vi "Tower_lamp.vi"(10 "DOs":bool[](array[boolean])=[TRUE, FALSE, FALSE, FALSE], 11 "Relay_Channel_OUT":T1[](array[typedef])) -> ()   [LabVIEW 2024, in "ADAM_DI.lvlib"]
uses:
  ADAM_DI.lvlib
  Relay_Enum_OUT.ctl
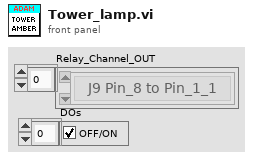
[diagram p1: front panel]
types:
  T1 = typedef "ADAM_DI.lvlib/Relay_Enum_OUT.ctl" = enum16{"J9 Pin_8 to Pin_1_1", "J9 Pin_8 to Pin_1_2", "J9 Pin_7 to Pin_1_1", "J9 Pin_7 to Pin_1_2", "J9 Pin_8 to Pin_7_1", "J9 Pin_8 to Pin_7_2", "J9 Pin_5 to Pin_1_1", "J9 Pin_5 to Pin_1_2", "J9 Pin_6 to Pin_1_1", "J9 Pin_6 to Pin_1_2", "J9 Pin_4 to Pin_1_1", "J9 Pin_4 to Pin_1_2", "J9 Pin_3 to Pin_1_1", "J9 Pin_3 to Pin_1_2", "PS(GND) to Pin1_1 J9", "PS(GND) to Pin1_2 J9", "PS(+14V) to Pin_3_1", "PS(+14V) to Pin_3_2", "PS(+12V) to Pin_4_1_ J9", "PS(+12V) to Pin_4_2_ J9", "PS(+12V) to Pin_5_1 J9", "PS(+12V) to Pin_5_2 J9", "PS(+12V) to Pin_6_1 J9", "PS(+12V) to Pin_6_2 J9", "Tower Amber", "Tower Red", "Tower Green", "Tower Buzzer", "PS(GND) to TP3_1", "PS(GND) to TP3_2", "PS(+14V) to TP19_1", "PS(+14V) to TP19_2", "PS(+12V) to TP33_1", "PS(+12V) to TP33_2", "PS(+12V) to TP38_1", "PS(+12V) to TP38_2", "PS(+12V) to TP40_1", "PS(+12V) to TP40_2", "TP19 (+14V) to TP3 (GND)_1", "TP19 (+14V) to TP3 (GND)_2", "TP1 (+14V) to TP3 (GND)_1", "TP1 (+14V) to TP3 (GND)_2", "TP2 (+5V) to TP3 (GND)_1", "TP2 (+5V) to TP3 (GND)_2", "TP6 (+14V) to TP9 (GND)_1", "TP6 (+14V) to TP9 (GND)_2", "TP7 (+3V8) to TP9 (GND)_1", "TP7 (+3V8) to TP9 (GND)_2", "TP11 (+14V) to TP13 (GND)_1", "TP11 (+14V) to TP13 (GND)_2", "TP12 (+3V) to TP13 (GND)_1", "TP12 (+3V) to TP13 (GND)_2", "TP5 (+3V3) to TP8 (GND)_1", "TP5 (+3V3) to TP8 (GND)_2", "TP48 (CAN_H) to TP3 (GND)_1", "TP48 (CAN_H) to TP3 (GND)_2", "TP41 (CAN_L) to TP3 (GND)_1", "TP41 (CAN_L) to TP3 (GND)_2", "TP48 (CAN_H) to TP41 (CAN_L)_1", "TP48 (CAN_H) to TP41 (CAN_L)_2", "TP38 (L_IND) to TP3 (GND)_1", "TP38 (L_IND) to TP3 (GND)_2", "TP40 (R_IND) to TP3 (GND)_1", "TP40 (R_IND) to TP3 (GND)_2", "TP33 (HB_CON) to TP3 (GND)_1", "TP33 (HB_CON) to TP3 (GND)_2", "TP19 (+14V) to TP34 (Q19-G)_1", "TP19 (+14V) to TP34 (Q19-G)_2", "TP55 (SW1) to TP3 (GND)_1", "TP55 (SW1) to TP3 (GND)_2", "TP56 (SW2) to TP3 (GND)_1", "TP56 (SW2) to TP3 (GND)_2", "TP66 WRT TP3 (GND)_1", "TP66 WRT TP3 (GND)_2", "TP19 WRT TP3_1", "TP19 WRT TP3_2", "TP1 WRT TP3_1", "TP1 WRT TP3_2", "TP2 WRT TP3_1", "TP2 WRT TP3_2", "TP7 WRT TP9_1", "TP7 WRT TP9_2", "TP12 WRT TP13_1", "TP12 WRT TP13_2", "TP5 WRT TP8_1", "TP5 WRT TP8_2", "TP22 WRT TP3_1", "TP22 WRT TP3_2", "TP52 WRT TP3(GND)_1", "TP52 WRT TP3(GND)_2", "TP50 WRT TP3(GND)_1", "TP50 WRT TP3(GND)_2", "TP51 WRT TP3(GND)_1", "TP51 WRT TP3(GND)_2"}
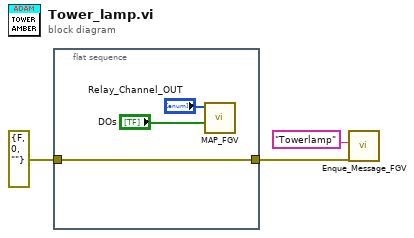
[diagram p0: block diagram]
diagram:
  n1 = flat-sequence {
    tunnel: errorcluster {"status"=FALSE, "code"=0, "source"=""} ("error out") -> [w5]
    tunnel: [w5] -> w2
    frame #0 {
      n2 = call "MAP_FGV.vi"("DOs"="DOs", "Relay_Channel_Out"="Relay_Channel_OUT") -> ()  [unwired: 7 in, 3 out]
    }
  }
  n3 = call "Enque_Message_FGV.vi"("error in (no error)"=w2, "Message"="Towerlamp") -> ()  [unwired: 9 in, 1 out]
